vi "Get All Albums.vi"(8 "error in (no error)":errorcluster, 11 "MusicLibrary in":refnum<class "MusicLibrary.lvclass">) -> (0 "error out":errorcluster, 2 "MusicLibrary":refnum<class "MusicLibrary.lvclass">, 3 "MusicLibrary out":refnum<class "MusicLibrary.lvclass">)   [LabVIEW 2015, in "MusicLibrary.lvclass"]
uses:
  MusicLibrary.lvclass
  MusicElementLibrary.lvclass/MusicElementLibrary.ctl
  Album/Album.lvclass
  MusicElement.lvclass
  MusicElementLibrary.lvclass
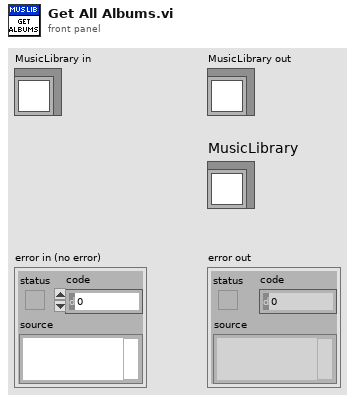
[diagram p1: front panel]
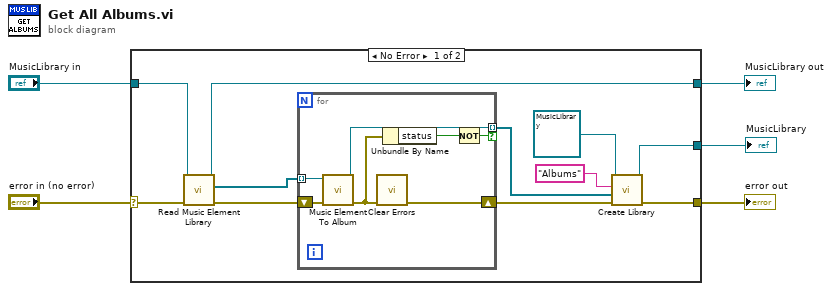
[diagram p0: block diagram]
diagram:
  n1 = case shown="No Error" "error in (no error)" {
    selector: "error in (no error)" -> [w16 w25]
    tunnel: [w8 w25] -> w4
    tunnel: [w13 w24] -> w2
    tunnel: "MusicLibrary in" -> [w14 w24]
    tunnel: [w6 _] -> w1
    frame No Error {
      n2 = call "Read Music Element Library.vi"("error in (no error)"=w16, "MusicElementLibrary in"=w14) -> ("error out"=w15:errorcluster, "Music Element Library"=w12:refnum<class "MusicElement.lvclass">[], "MusicElementLibrary out"=w13:refnum<class "MusicLibrary.lvclass">)  [unwired: 7 in]
      n3 = for {
        shift-right: [w17] -> w11
        shift-left: w15 -> [w23]
        tunnel: w12 -> [w22] mode=indexing
        tunnel: [w21] -> w10 mode=indexing if=w18
        n4 = call "Music Element To Album.vi"("error in (no error)"=w23, "MusicElement"=w22) -> ("error out"=w20:errorcluster, "Album"=w21:refnum<class "Album.lvclass">)  [unwired: 8 in]
        n5 = call <vilib>:"Clear Errors.vi"("error in (no error)"=w20) -> ("error out"=w17:errorcluster)  [unwired: 5 in, 1 out]
        n6 = Unbundle By Name(w20) -> ("status"=w19:bool)
        n7 = Not(x=w19) -> (.not. x?=w18:bool)
      }
      n8 = call "Create Library.vi"("error in (no error)"=w11, "Music Element Library"=w10, "Name"="Albums", "MusicElementLibrary in"=refnum<class "MusicLibrary.lvclass"> refnum ("MusicLibrary.lvclass")) -> ("error out"=w8:errorcluster, "MusicElementLibrary out"=w6:refnum<class "MusicLibrary.lvclass">)  [unwired: 6 in]
    }
    frame Error {
    }
  }
  "error out" <- w4
  "MusicLibrary out" <- w2
  "MusicLibrary" <- w1
